vi "Destroy Data Channels.vi"(8 "error in":errorcluster, 11 "Node in":refnum<class "BTSTemplateTest.lvclass">) -> (0 "error out":errorcluster, 3 "Node out":refnum<class "BTSTemplateTest.lvclass">)   [LabVIEW 2023, in "BTSTemplateTest.lvlib" / "BTSTemplateTest.lvclass"]
uses:
  BTSTemplateTest.lvclass
  BTSTemplateTest.lvclass/BTSTemplateTest.ctl
  <vilib>/ADAS Replay HIL/AdasHilServices/AdasHilServices Fill In Error Info Ex.vi
  <vilib>/BTS Capabilities/Cycler/Cycler.lvclass
  C:/Program Files/NI/LVAddons/btscapabilities/1/vi.lib/BTS Capabilities/Capability/Capability.lvclass
  C:/Program Files/NI/LVAddons/btscapabilities/1/vi.lib/BTS Capabilities/Cycler/Cycler.lvclass
  <vilib>/BTS Capabilities/Control Mode/Control Mode.lvclass
  C:/Program Files/NI/LVAddons/btscapabilities/1/vi.lib/BTS Capabilities/Control Mode/Control Mode.lvclass
  <vilib>/BTS Capabilities/Current/Current Control.lvclass
  C:/Program Files/NI/LVAddons/btscapabilities/1/vi.lib/BTS Capabilities/Current/Current Control.lvclass
  <vilib>/BTS Capabilities/Current Limits/Current Limits.lvclass
  C:/Program Files/NI/LVAddons/btscapabilities/1/vi.lib/BTS Capabilities/Current Limits/Current Limits.lvclass
  <vilib>/BTS Capabilities/Voltage/Voltage Control.lvclass
  C:/Program Files/NI/LVAddons/btscapabilities/1/vi.lib/BTS Capabilities/Voltage/Voltage Control.lvclass
  <vilib>/BTS Capabilities/Voltage Limits/Voltage Limits.lvclass
  C:/Program Files/NI/LVAddons/btscapabilities/1/vi.lib/BTS Capabilities/Voltage Limits/Voltage Limits.lvclass
  <vilib>/BTS Capabilities/Power/Power Control.lvclass
  C:/Program Files/NI/LVAddons/btscapabilities/1/vi.lib/BTS Capabilities/Power/Power Control.lvclass
  <vilib>/BTS Capabilities/Power Limits/Power Limits.lvclass
  C:/Program Files/NI/LVAddons/btscapabilities/1/vi.lib/BTS Capabilities/Power Limits/Power Limits.lvclass
  <vilib>/BTS Capabilities/Capability/Capability.lvclass
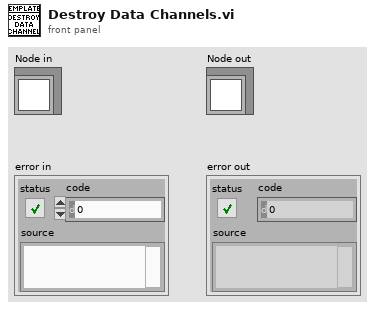
[diagram p1: front panel]
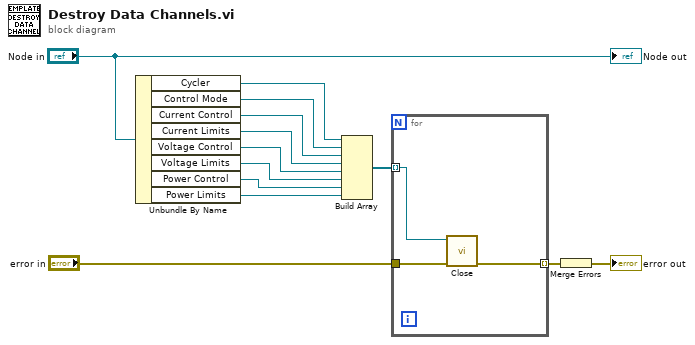
[diagram p0: block diagram]
diagram:
  n1 = Unbundle By Name("Node in") -> ("Cycler"=w12:refnum<class "Cycler.lvclass">, "Control Mode"=w11:refnum<class "Control Mode.lvclass">, "Current Control"=w10:refnum<class "Current Control.lvclass">, "Current Limits"=w9:refnum<class "Current Limits.lvclass">, "Voltage Control"=w8:refnum<class "Voltage Control.lvclass">, "Voltage Limits"=w7:refnum<class "Voltage Limits.lvclass">, "Power Control"=w6:refnum<class "Power Control.lvclass">, "Power Limits"=w5:refnum<class "Power Limits.lvclass">)
  n2 = Build Array(w12, w11, w10, w9, w8, w7, w6, w5) -> (w2:refnum<class "Capability.lvclass">[])
  n3 = for {
    tunnel: w2 -> [w16] mode=indexing
    tunnel: "error in" -> [w15]
    tunnel: [w14] -> w4 mode=indexing
    n4 = call-dynamic "Close.vi"("error in (no error)"=w15, "Capability in"=w16) -> ("error out"=w14:errorcluster)  [unwired: 8 in, 1 out]
  }
  n5 = Merge Errors(w4) -> (→"error out":errorcluster)
  "Node out" <- "Node in"
